vi "GeneCfgFile.vi"(4 "error in":errorcluster caption="entrée d'erreur (pas d'erreur)", 7 "NomProjet":string) -> (0 "sortie d'erreur":errorcluster, 3 "NomProjetOut":string)   [LabVIEW 2015]
uses:
  DefDeType/WhichPath.ctl
  DefDeType/WBridgeChannels.ctl
  DefDeType/VoltageChannels.ctl
  DefDeType/Configuration.ctl
  DefDeType/ConfigTotale.ctl
panel:
  out "ConfigTotale":T1
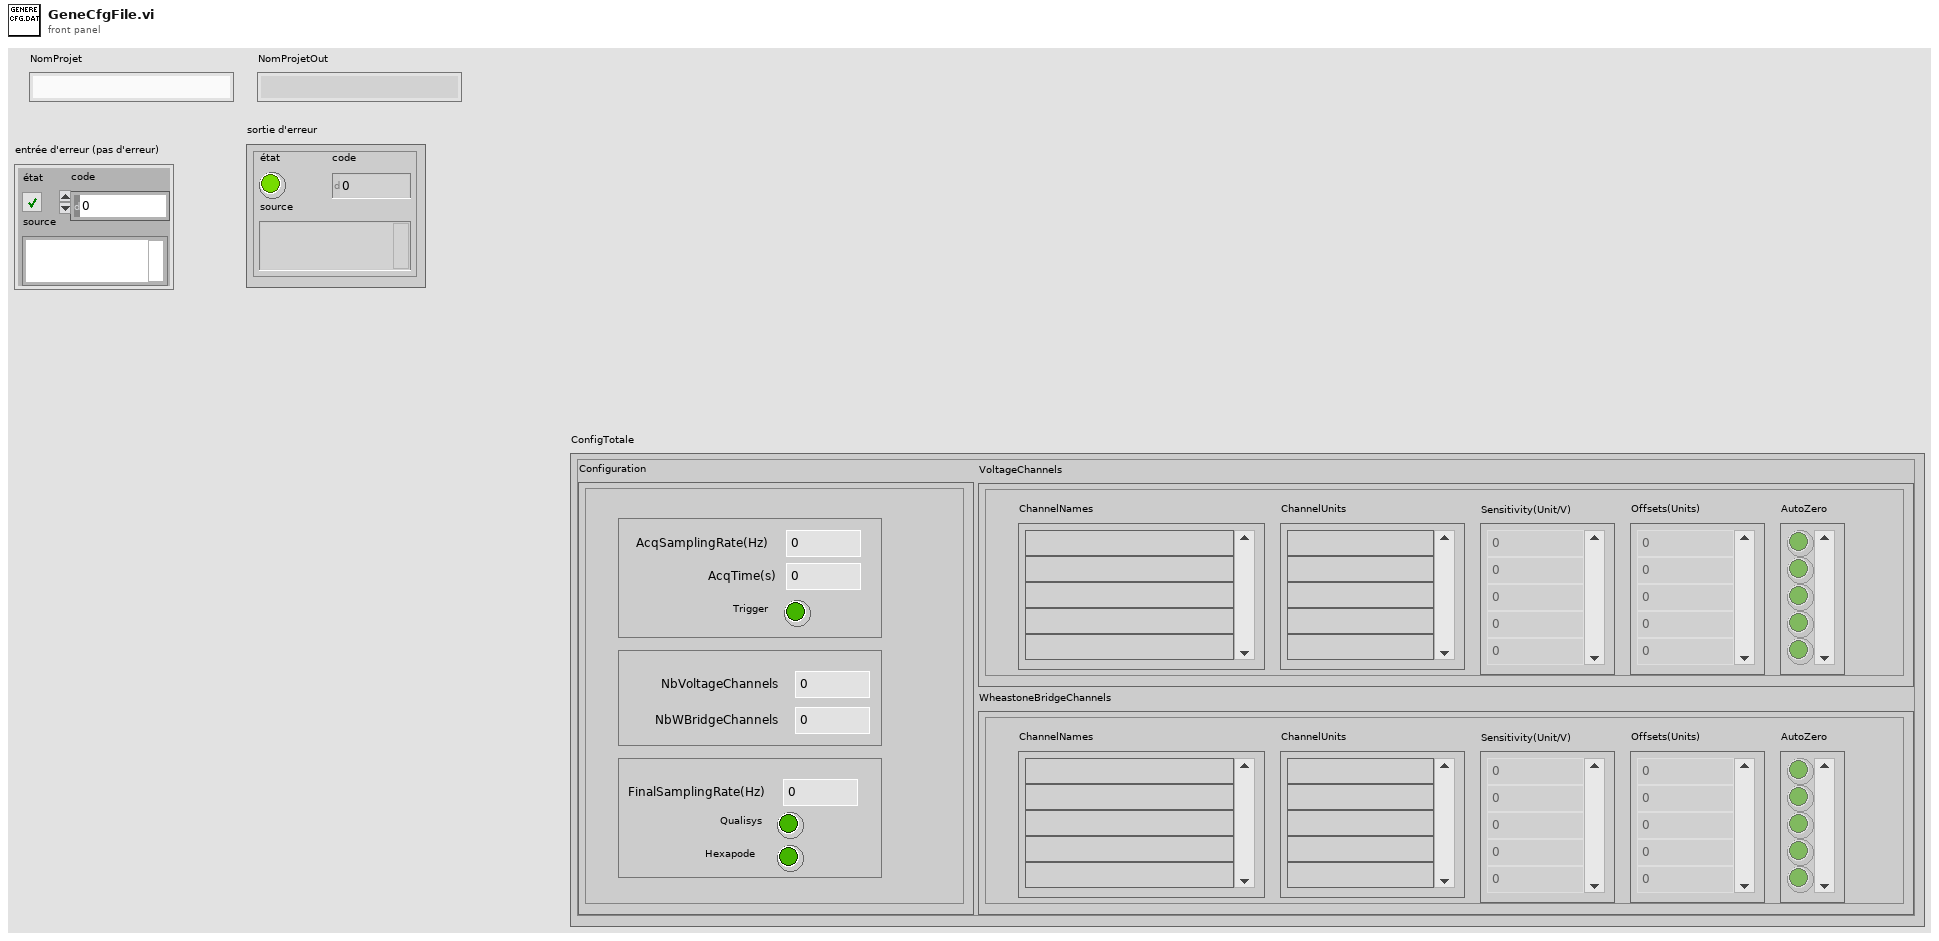
[diagram p1: front panel]
types:
  T1 = typedef "ConfigTotale.ctl" = cluster{"Configuration":T2, "VoltageChannels":T3, "WheastoneBridgeChannels":T4}
  T2 = typedef "Configuration.ctl" = cluster{"AcqSamplingRate(Hz)":u32, "AcqTime(s)":u32, "Trigger":bool, "NbVoltageChannels":u32, "NbWBridgeChannels":u32, "Qualisys":bool, "Hexapode":bool, "FinalSamplingRate(Hz)":u32}
  T3 = typedef "VoltageChannels.ctl" = cluster{"ChannelNames":string[], "Sensitivity(Unit/V)":dbl[], "AutoZero":bool[], "ChannelUnits":string[], "Offsets(Units)":dbl[]}
  T4 = typedef "WBridgeChannels.ctl" = cluster{"ChannelNames":string[], "Sensitivity(Unit/V)":dbl[], "AutoZero":bool[], "ChannelUnits":string[], "Offsets(Units)":dbl[]}
  T5 = enum16{"open", "replace", "create", "open or create", "replace or create", "replace or create with confirmation"}
  T6 = typedef "WhichPath.ctl" = enum16{"DossierProjet", "Config", "Meas", "MeasSuitCase", "MeasOnBoard", "MeasQualisys", "MeasTDMS", "MeasHexapode", "Fig", "Res"}
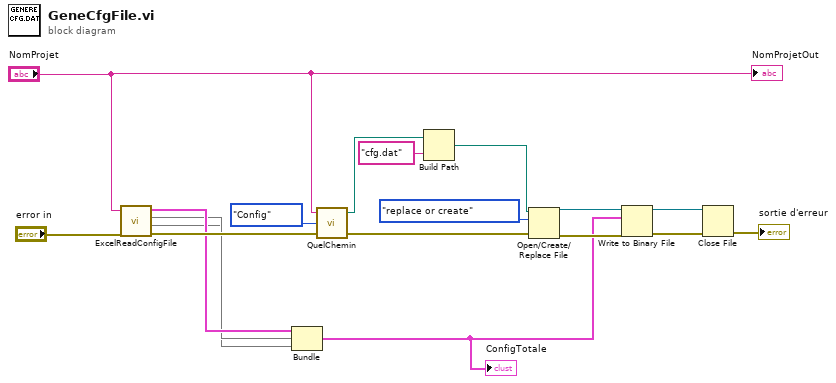
[diagram p0: block diagram]
diagram:
  n1 = call "ExcelReadConfigFile.vi"("NomProjet"="NomProjet", "error in (no error)"="error in") -> ("ConfigurationTotale"=w6:T1, 4:w5, 5:w4, "error out"=w15:errorcluster)  [unwired: 1 in]
  n2 = Bundle("ConfigurationTotale"=w6, w5, w4) -> (w1:cluster{"ConfigurationTotale":T1, void, void})  [unwired: 1 in]
  "ConfigTotale" <- w1
  n3 = call "QuelChemin.vi"("Entrée d'erreur"=w15, "WhichPath?"=WhichPath."Config", "NomProjet"="NomProjet") -> ("Sortie d'erreur"=w12:errorcluster, "SurDisqueLocal"=w14:path)  [unwired: 1 out]
  n4 = Build Path(base path=w14, name or relative path="cfg.dat" ("nom ou chemin relatif")) -> (appended path=w11:path)
  n5 = Open/Create/Replace File(file path (use dialog)=w11, error in=w12, operation (0:open)=T5."replace or create" ("opération (0 : open)")) -> (refnum out=w7:refnum<file>, error out=w9:errorcluster)  [unwired: 3 in, 1 out]
  n6 = Write to Binary File(file (use dialog)=w7, data=w1, error in=w9) -> (refnum out=w3:refnum<file>, error out=w8:errorcluster)  [unwired: 3 in, 1 out]
  n7 = Close File(refnum=w3, error in=w8) -> (error out=→"sortie d'erreur":errorcluster)  [unwired: 1 out]
  "NomProjetOut" <- "NomProjet"
